vi "Dashboard Main.vi"() -> ()   [LabVIEW 2020]
uses:
  <vilib>/event_ctls.llb/eventvkey.ctl
  <vilib>/Rock Robotics/Network Tables/NT Read Numeric Array.vi
  <vilib>/Rock Robotics/Network Tables/NT Read Boolean.vi
  <vilib>/Rock Robotics/WPI/Dashboard/WPI_DashboardLogging Global.vi
panel:
  in  "Camera Settings Right":T1={"Frame Rate"=30, "Compression"=30, "Size"=1, "DB Camera Config"=FALSE} {"Frame Rate" scale=1.0..30.0; "Compression" scale=100.0..-1.0; "Size" items=["640x480", "320x240", "160x120"]}
  in  "Camera Name Right":string(combo)="No Camera Selection"
  out "Camera Perf":string
  in  "Camera Settings":T1={"Frame Rate"=30, "Compression"=30, "Size"=1, "DB Camera Config"=FALSE} {"Frame Rate" scale=1.0..30.0; "Compression" scale=100.0..-1.0; "Size" items=["640x480", "320x240", "160x120"]}
  in  "TCP":refnum<k5>
  in  "Rec Mode":enum32{"Stop", "Record", "Playback"}(radio)
  out "Robot IP":string
  out "Image Message":string="Timeout in Camera Communications"
  in  "Dashboard Tab":T2(tab)
  out "Reverse":bool
  out "Speed Modifer":dbl
  in  "Select Auto":string(combo)="Select Autonomous ..."
  out "NT Connection":bool
  out "JS1 Z":dbl(slide) scale=-1.0..1.0 scale format="%#_2e"
  out "JS1 Graph":cluster{"X":dbl, "Y":dbl}[](graph)
  out "JS1 Buttons":T3
  out "JS2 Z":dbl(slide) scale=-1.0..1.0 scale format="%#_2e"
  out "JS2 Graph":cluster{"X":dbl, "Y":dbl}[](graph)
  out "JS2 Buttons":T3
  out "Mode":T4(ring)=enum."Auto Disabled"
  out "Right Camera Perf":cluster{"Bandwidth (Mbps)":dbl, "FPS":dbl}
  out "Camera Image Right":T5(plugin-control)
  in  "DB/String 9":string
  in  "DB/String 8":string
  in  "DB/String 7":string
  in  "DB/String 6":string
  in  "DB/String 5":string
  in  "DB/String 4":string
  in  "DB/String 3":string
  in  "DB/String 2":string
  in  "DB/String 1":string
  in  "DB/String 0":string
  in  "DB/Slider 0":dbl(slide) scale=0.0..5.0
  in  "DB/Slider 1":dbl(slide) scale=0.0..5.0
  in  "DB/Slider 2":dbl(slide) scale=0.0..5.0
  in  "DB/Slider 3":dbl(slide) scale=0.0..5.0
  out "DB/LED 3":bool
  out "DB/LED 2":bool
  out "DB/LED 1":bool
  out "DB/LED 0":bool
  in  "DB/Button 3":bool
  in  "DB/Button 2":bool
  in  "DB/Button 1":bool
  in  "DB/Button 0":bool caption="New Name"
  in  "Test Slider":dbl(slide) scale=0.0..100.0 scale format="%#_3g"
  in  "On/Off":bool caption="Solenoid"
  in  "Test Name":u16(ring) items=["Select the test to run..."]
  in  "Test Tree":string(tree)
  in  "Motor":cluster{"Value":dbl, "Enable":bool} {"Value" scale=-1.0..1.0 scale format="%#_3g"}
  out "Progress":T6 {"Test Progress" scale=0.0..100.0}
  in  "Rev/Fwd":cluster{"Forward":bool, "Reverse":bool}
  in  "Test Ring":u16(ring) items=["Monochrome", "Color"]
  in  "CheckList":i32(listbox)
  out "Tree":string(tree)
  out "Camera Image":T5(plugin-control)
  out "Background":bool
  in  "Camera Name":string(combo)="No Camera Selection"
  # "HW"
  # "HW"
  # "Joysticks"
  # "This tab is a great place for autonomous settings and robot-specific values.\nPlace controls and indicators inside this tab and match name to\nDashboard Variables on robot. You can also delete this comment."
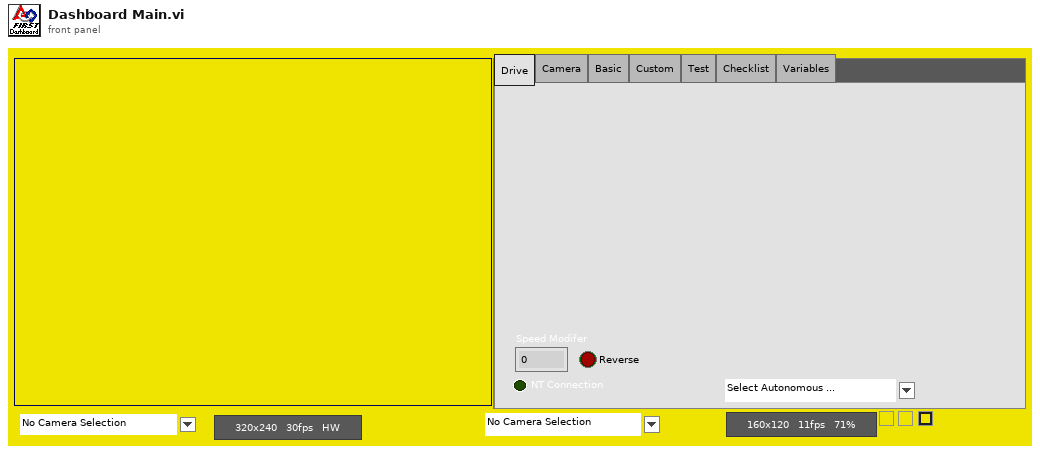
[diagram p1: front panel]
types:
  T1 = cluster{"Frame Rate":i32, "Compression":i32, "Size":u16, "DB Camera Config":bool}
  T2 = enum32{"Drive", "Camera", "Basic", "Custom", "Test", "Checklist", "Variables"}
  T3 = cluster{bool, bool, bool, bool, bool, bool, bool, bool, bool, bool, bool, bool}
  T4 = enum8{"Tele-Op Disabled", "Tele-Op Enabled", "Auto Disabled", "Auto Enabled", "Test Disabled", "Test Enabled", "Disconnected", "No Code", "E-Stop"}
  T5 = typedef "IMAQ Image.ctl" = refnum<image>
  T6 = cluster{"Test Progress":u8, "Test Progress Text":string}
  T7 = cluster{"Save Path":path, "Interval (s)":dbl, "Keep":i32}
  T8 = enum32{"Drive", "Camera", "Basic", "Custom", "Test", "Commands", "Checklist", "Variables"}
  T9 = typedef "Image Type" = u32
  T10 = cluster{"Error Strings":string, "Disable Counts":cluster{u16, u16}, "Rail Faults":cluster{u16, u16, u16}, "Robot IP":string, "DB Mode":u8, "Event Info":cluster{"Name":string, "Type":u8, "Number":u16, "Replay":u8}}
  T11 = cluster{"Storage":cluster{"Disk Free":u64, "RAM Block":u32, "RAM free":u32}, "CPU Utilization":cluster{"CPU % ISR":sgl, "CPU % Time Crit":sgl, "CPU % Timed Str":sgl, "CPU % High":sgl, "CPU % Above":sgl, "CPU % Normal":sgl, "CPU % Low":sgl}, "CAN":cluster{"% Bus Utilization":sgl, "Bus Off Cnt":u32, "TX_FIFO Full Cnt":u32, "Receive Error Cnt":u8, "Transmit Error Cnt":u8}, "HID":cluster{"HID Outputs":u32, "Rumble Low":u16, "Rumble High":u16}[]}
  T12 = cluster{"Status bits":cluster{"Test Mode":bool, "Autonomous":bool, "Enabled":bool, "Code Start":bool, "Brownout":bool, "Reserved 2":bool, "Reserved 3":bool, "E-Stop":bool}, "Code Trace":cluster{"Disabled":bool, "TeleOp":bool, "Auto":bool, "Test":bool}, "Controller Type":enum16{"unknown", "cRIO", "roboRio"}, "Code?":enum16{"unknown", "noCode", "code"}, "Battery V":dbl}
  T13 = cluster{"Control Bits":cluster{"TestMode":bool, "Autonomous":bool, "Enabled":bool, "FMS Present":bool, bool, bool, bool, "E-Stop":bool}, "Team Station ":u8, "Countdown":sgl, "Joystick Values":cluster{"Axes":dbl[], "Buttons":bool[], "POVs":i16[]}[]}
  T14 = cluster{"Axes":dbl[], "Buttons":bool[], "POVs":i16[]}[]
  T15 = cluster{"Axes":dbl[], "Buttons":bool[], "POVs":i16[]}
  T16 = cluster{"Buttons[0]":bool, "Buttons[1]":bool, "Buttons[2]":bool, "Buttons[3]":bool, "Buttons[4]":bool, "Buttons[5]":bool, "Buttons[6]":bool, "Buttons[7]":bool, "Buttons[8]":bool, "Buttons[9]":bool, "Buttons[10]":bool, "Buttons[11]":bool}
  T17 = cluster{"Camera Image":refnum<vi>, "Dashboard Tab":refnum<vi>, "Background":refnum<vi>, "Rec Mode":refnum<vi>, "Test Slider":refnum<vi>, "On/Off ":refnum<vi>, "Test Ring":refnum<vi>, "Rev/Fwd":refnum<vi>, "Test Name":refnum<vi>, "Motor":refnum<vi>, "Progress":refnum<vi>, "CheckList":refnum<vi>, "Tree":refnum<vi>, "Test Tree":refnum<vi>, "Camera Settings":refnum<vi>, "Camera Name":refnum<vi>, "Camera Perf":refnum<vi>, "Camera Settings Right":refnum<vi>, "Camera Name Right":refnum<vi>, "Camera Image Right":refnum<vi>}
  T18 = cluster{"Global Rectangle":i32[], "Contours":cluster{"Contour Type":u32, "ROI Type":u32, "Points":i32[]}[]}
  T19 = cluster{"Camera Name":string, string, "Saved DB Images Info":cluster{"Save Path":path, "Interval (s)":dbl, "Keep":i32}}
  T20 = cluster{"Camera Name Right":string, string, "Saved DB Images Info":cluster{"Save Path":path, "Interval (s)":dbl, "Keep":i32}}
  T21 = cluster{"Operation":enum16{"Update", "Clear"}, "Color Box":u32}[]
  T22 = typedef "eventvkey.ctl" = enum16{"ASCII", "Enter", "Return", "Shift", "Ctrl", "Alt", "Cmd", "Opt", "Caps", "NumLock", "Clear", "Break", "Up", "Down", "Left", "Right", "Insert", "Delete", "Home", "End", "PageUp", "PageDown", "Escape", "Help", "Pause", "ScrollLock", "F1", "F2", "F3", "F4", "F5", "F6", "F7", "F8", "F9", "F10", "F11", "F12", "F13", "F14", "F15", "F16", "F17", "F18", "F19", "F20", "F21", "F22", "F23", "F24", "Play", "VolumeUp", "VolumeDown", "Mute", "Two Byte Char"}
  T23 = cluster{"Image Size":bool, "Image Type":bool, "Pixel Value":bool, "ROI Information":bool, "Zoom Factor":bool}
  T24 = cluster{"Operation":enum16{"Update", "Clear"}, "Color Box":u32}
  T25 = cluster{"Shift":bool, "Ctrl":bool, "Alt":bool, "Cmd":bool, "Opt":bool}
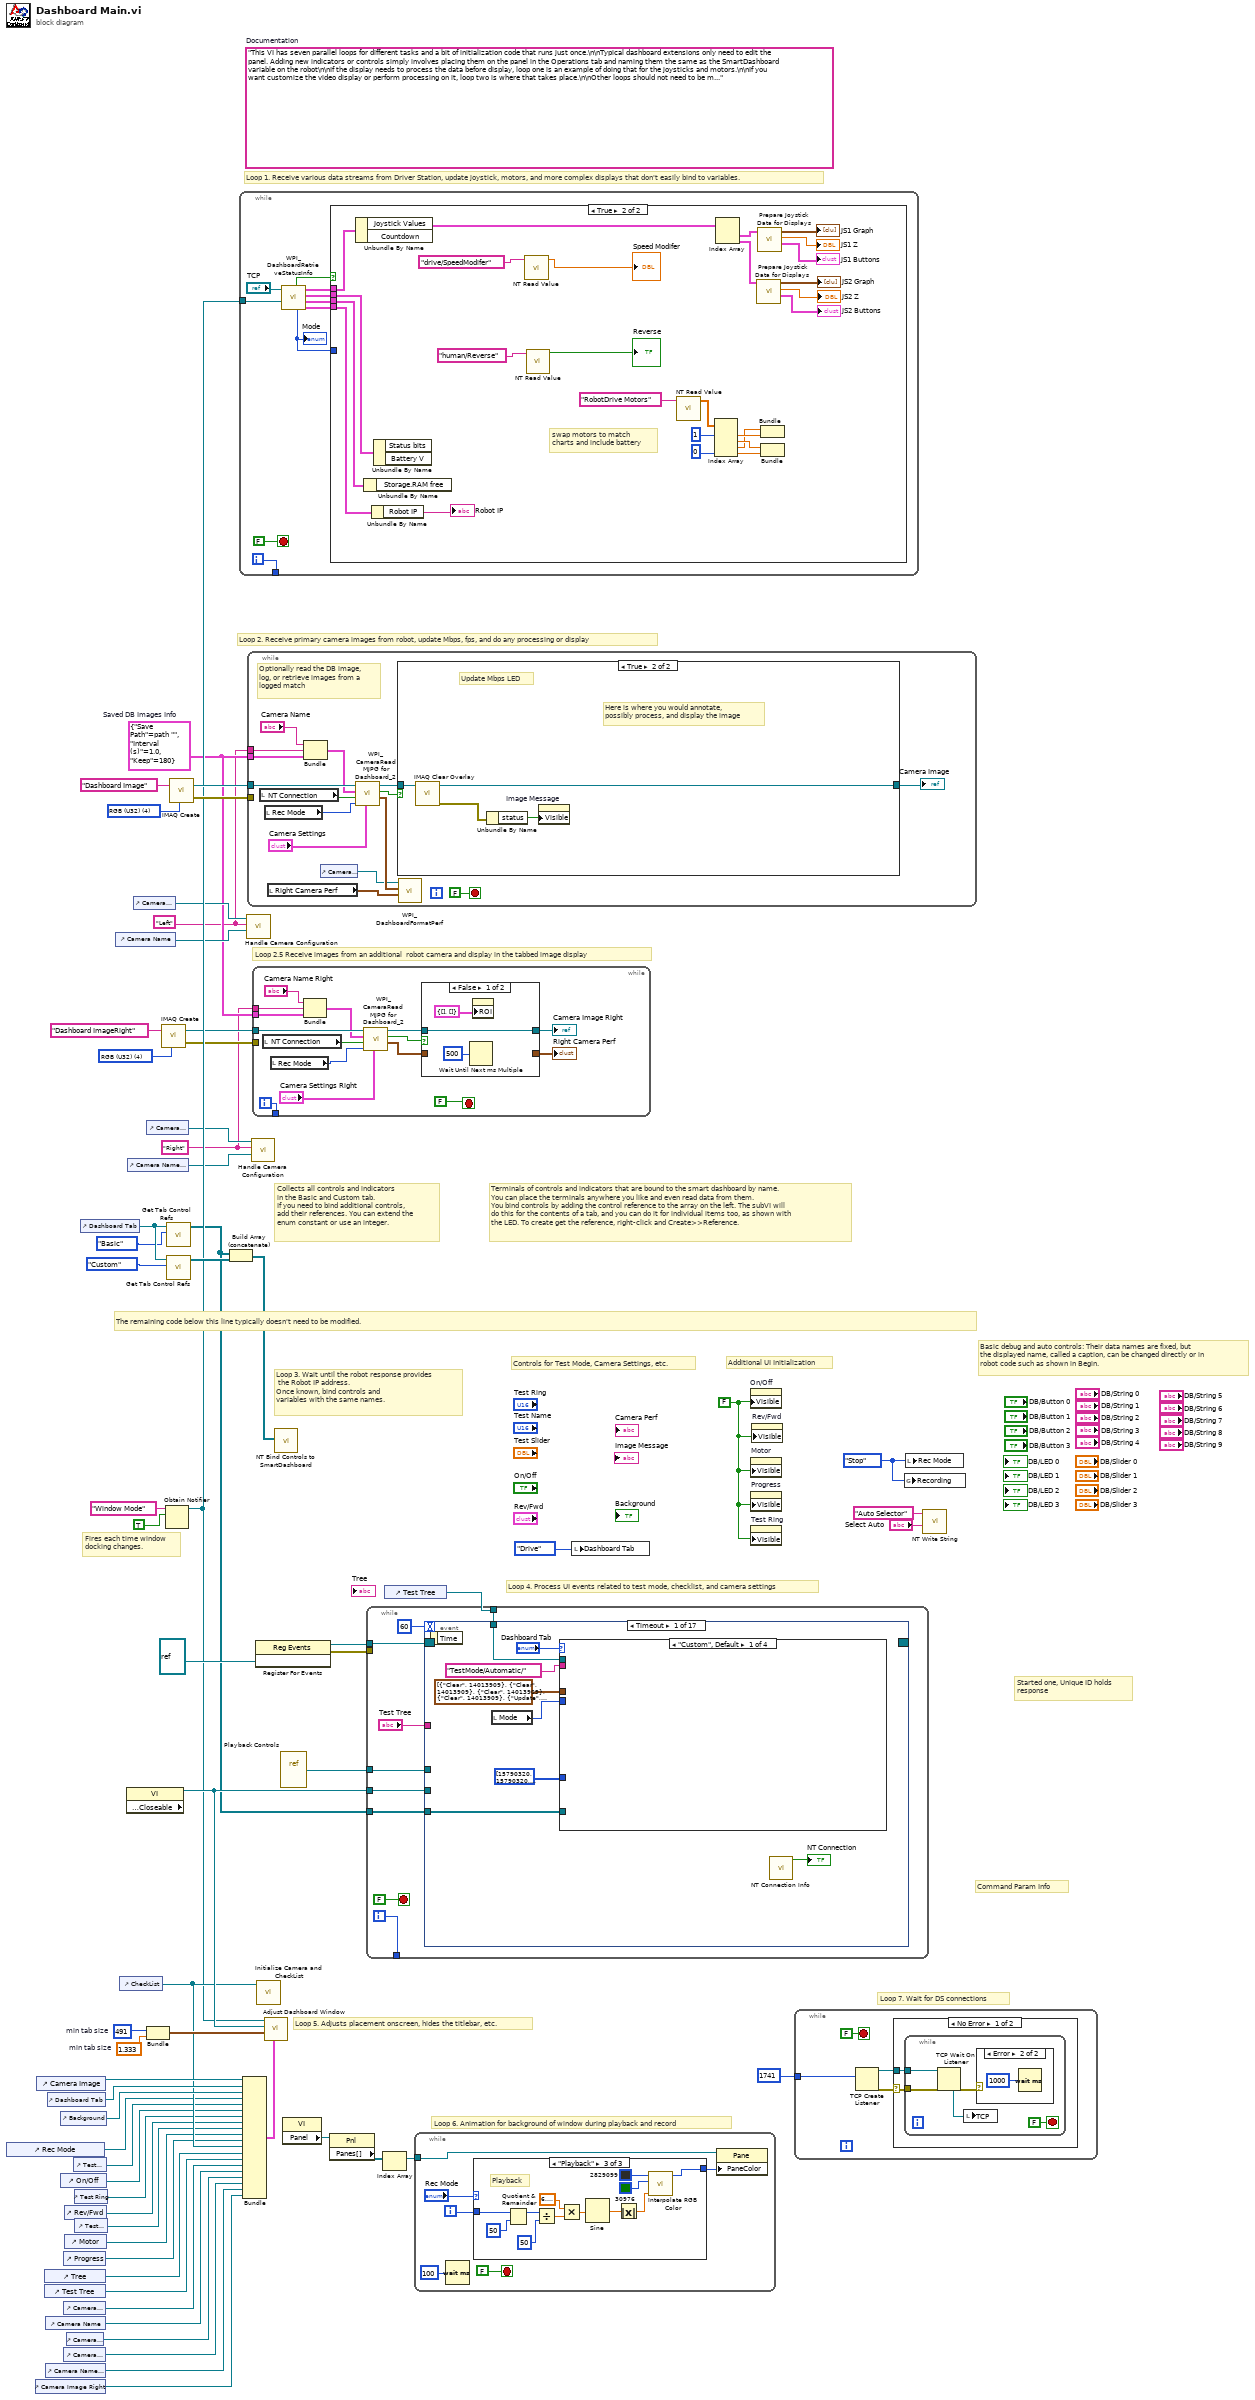
[diagram p0: block diagram]
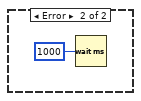
[diagram p4: hidden frame]
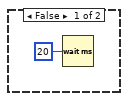
[diagram p5: hidden frame]
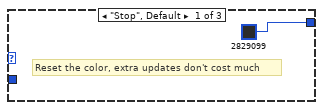
[diagram p6: hidden frame]
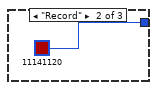
[diagram p7: hidden frame]
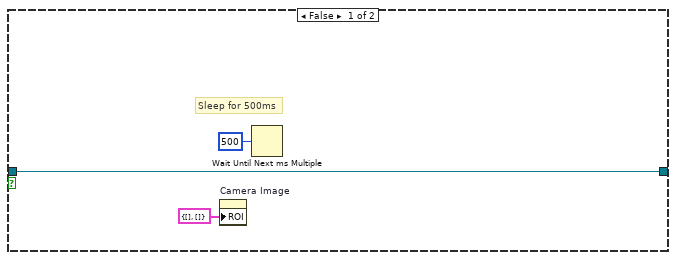
[diagram p8: hidden frame]
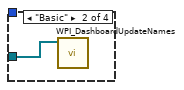
[diagram p9: hidden frame]
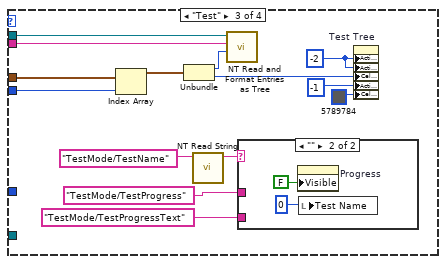
[diagram p10: hidden frame]
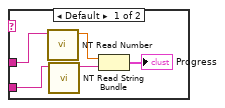
[diagram p11: hidden frame]
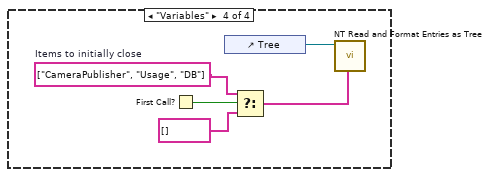
[diagram p12: hidden frame]
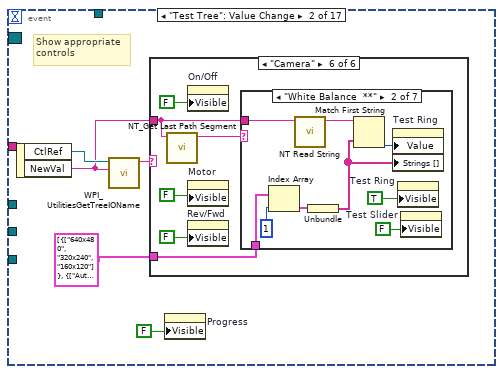
[diagram p13: hidden frame]
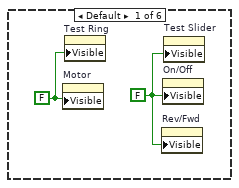
[diagram p14: hidden frame]
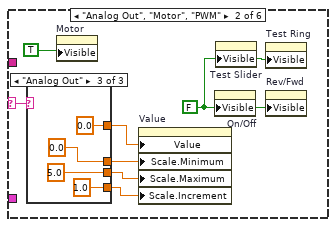
[diagram p15: hidden frame]
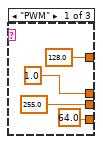
[diagram p16: hidden frame]
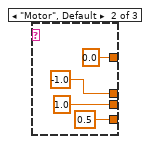
[diagram p17: hidden frame]
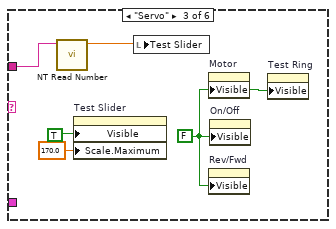
[diagram p18: hidden frame]
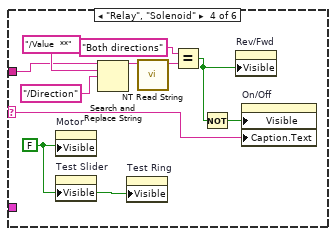
[diagram p19: hidden frame]
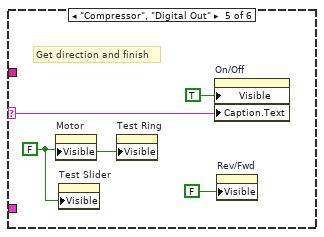
[diagram p20: hidden frame]
diagram:
  w3 = T7 {"Save Path"=path "", "Interval (s)"=1.0, "Keep"=180}  # Saved DB Images Info
  w2 = "Right"
  w1 = "Left"
  w13 = T9 4 items=["Grayscale (U8)", "Grayscale (I16)", "Grayscale (SGL)", "Complex (CSG)", "RGB (U32)", "HSL (U32)", "RGB (U64)"] ("Image Type")
  w42 = 491  # min tab size
  w41 = 1.333  # min tab size
  w49 = enum32{"Stop", "Record", "Playback"}."Stop" ("Rec Mode")
  w26 = FALSE ("Visible")
  (unwired) "This VI has seven parallel loops for different tasks and a bit of initialization code that runs just once.\n\nTypical dashboard extensions only need to edit the panel. Adding new indicators or controls simply involves placing them on the panel in the Operations tab and naming them the same as the SmartDashboard variable on the robot\n\nIf the display needs to process the data before display, loop one is an example of doing that for the joysticks and motors.\n\nIf you want customize the video display or perform processing on it, loop two is where that takes place.\n\nOther loops should not need to be modified. They are pretty standard, and document the task they perform."  # Documentation
  w63 = T9 4 items=["Grayscale (U8)", "Grayscale (I16)", "Grayscale (SGL)", "Complex (CSG)", "RGB (U32)", "HSL (U32)", "RGB (U64)"] ("Image Type")
  # "Loop 2.5 Receive images from an additional  robot camera and display in the tabbed image display"
  # "Command Param Info"
  # "Started one, Unique ID holds\nresponse"
  # "Loop 7. Wait for DS connections"
  # "Basic debug and auto controls: Their data names are fixed, but\nthe displayed name, called a caption, can be changed directly or in\nrobot code such as shown in Begin."
  # "Controls for Test Mode, Camera Settings, etc."
  # "Additional UI Initialization"
  # "Loop 6. Animation for background of window during playback and record"
  # "Fires each time window\ndocking changes."
  # "Collects all controls and indicators\nin the Basic and Custom tab.\nIf you need to bind additional controls,\nadd their references. You can extend the\nenum constant or use an integer."
  # "The remaining code below this line typically doesn't need to be modified."
  # "Loop 4. Process UI events related to test mode, checklist, and camera settings"
  # "Terminals of controls and indicators that are bound to the smart dashboard by name.\nYou can place the terminals anywhere you like and even read data from them.\nYou bind controls by adding the control reference to the array on the left. The subVI will\ndo this for the contents of a tab, and you can do it for individual items too, as shown with\nthe LED. To create get the reference, right-click and Create>>Reference."
  # "Loop 3. Wait until the robot response provides\n the Robot IP address.\nOnce known, bind controls and\nvariables with the same names."
  # "Loop 5. Adjusts placement onscreen, hides the titlebar, etc."
  # "Loop 1. Receive various data streams from Driver Station, update joystick, motors, and more complex displays that don't easily bind to variables."
  # "Loop 2. Receive primary camera images from robot, update Mbps, fps, and do any processing or display"
  n1 = control-ref of="Rec Mode"() -> (w32:refnum<vi>)
  n2 = control-ref of="Camera Image Right"() -> (w6:refnum<vi>)
  n3 = control-ref of="Camera Image"() -> (w44:refnum<vi>)
  n4 = control-ref of="Tree"() -> (w36:refnum<vi>)
  n5 = control-ref of="Test Tree"() -> (w35:refnum<vi>)
  n6 = control-ref of="Camera Name"() -> (w19:refnum<vi>)
  n7 = control-ref of="Camera Name Right"() -> (w7:refnum<vi>)
  n8 = control-ref of="Dashboard Tab"() -> (w43:refnum<vi>)
  n9 = control-ref of="Background"() -> (w39:refnum<vi>)
  n10 = control-ref of="On/Off"() -> (w30:refnum<vi>)
  n11 = control-ref of="Progress"() -> (w27:refnum<vi>)
  n12 = control-ref of="Camera Settings"() -> (w20:refnum<vi>)
  n13 = control-ref of="Camera Settings Right"() -> (w8:refnum<vi>)
  n14 = control-ref of="Rev/Fwd"() -> (w28:refnum<vi>)
  n15 = control-ref of="Motor"() -> (w33:refnum<vi>)
  n16 = control-ref of="Camera Perf"() -> (w18:refnum<vi>)
  n17 = control-ref of="Test Slider"() -> (w31:refnum<vi>)
  n18 = control-ref of="Test Ring"() -> (w29:refnum<vi>)
  n19 = control-ref of="Test Name"() -> (w34:refnum<vi>)
  n20 = control-ref of="Dashboard Tab"() -> (w47:refnum<vi>)
  n21 = control-ref of="Camera Name"() -> (w21:refnum<vi>)
  n22 = control-ref of="CheckList"() -> (w37:refnum<vi>)
  n23 = property class="VI" props=["Front Panel.Closeable"]() -> (reference out=w48:refnum<vi>)  [unwired: 2 in, 2 out]
  n24 = control-ref of="Camera Name Right"() -> (w9:refnum<vi>)
  n25 = control-ref of="Camera Settings"() -> (w22:refnum<vi>)
  n26 = control-ref of="Camera Settings Right"() -> (w10:refnum<vi>)
  n27 = Bundle("min tab size"=w42, "min tab size"=w41) -> (w40:cluster{"min tab size":i32, "min tab size":dbl})  [unwired: 1 in]
  n28 = call "IMAQ Create"("Image Name"="Dashboard ImageRight", "Image Type"=w13) -> ("New Image"=w12:T5, "error out"=w11:errorcluster)  [unwired: 2 in, 1 out]
  n29 = Obtain Notifier(name (unnamed)="Window Mode", notification data type=TRUE) -> (notifier out=w25:refnum<notifier>)  [unwired: 2 in, 2 out]
  n30 = call <vilib>:"Get Tab Control Refs.vi"("Page Index"=T8."Basic" ("Dashboard Tab"), "TabControl in"=w47) -> ("ControlsOnPage"=w17:refnum<vi>[])  [unwired: 9 in]
  n31 = call <vilib>:"Get Tab Control Refs.vi"("Page Index"=T8."Custom" ("Dashboard Tab"), "TabControl in"=w47) -> ("ControlsOnPage"=w46:refnum<vi>[])  [unwired: 9 in]
  n32 = call "IMAQ Create"("Image Name"="Dashboard Image", "Image Type"=w63) -> ("New Image"=w61:T5, "error out"=w60:errorcluster)  [unwired: 2 in, 1 out]
  n33 = Build Array (concatenate)(w17, w46) -> (w45:refnum<vi>[])
  n34 = while {
    tunnel: [w72] -> _
    tunnel: w25 -> [w64]
    i -> [w72]
    stop <- FALSE stop-if-true
    n35 = call <vilib>:"WPI_DashboardRetrieveStatusInfo.vi"("Window Mode Notifier"=w64, "TCP Cnx"="TCP") -> ("Power and Errors"=w67:T10, "Robot Metrics"=w70:T11, "Status Info"=w71:T12, "Control Info"=w68:T13, "Robot Mode"=w66:T4, "Process?"=w69:bool)  [unwired: 4 in]
    "Mode" <- w66
    n36 = case shown="True" w69 {
      tunnel: w71 -> [_ w100]
      tunnel: w70 -> [_ w99]
      tunnel: w68 -> [_ w98]
      tunnel: w67 -> [_ w97]
      tunnel: w66 -> [_ _]
      frame False {
        n37 = Wait (ms)(milliseconds to wait=u32 20) -> ()  [unwired: 1 out]
      }
      frame True {
        # "swap motors to match\ncharts and include battery"
        n38 = Unbundle By Name(w98) -> ("Joystick Values"=w90:T14)  [unwired: 1 out]
        n39 = Unbundle By Name(w99) -> ()  [unwired: 1 out]
        n40 = Unbundle By Name(w97) -> ("Robot IP"=→"Robot IP":string)
        n41 = Unbundle By Name(w100) -> ()  [unwired: 2 out]
        n42 = call-poly <vilib>:"NT Read Value.vi"("name"="drive/SpeedModifer") -> ("value"=→"Speed Modifer":dbl)  [unwired: 8 in, 2 out]
        n43 = call-poly <vilib>:"NT Read Value.vi"("name"="human/Reverse") -> ("value"=→"Reverse":bool)  [unwired: 8 in, 2 out]
        n44 = call-poly <vilib>:"NT Read Value.vi"("name"="RobotDrive Motors" ("Name")) -> ("value"=w80:dbl[])  [unwired: 8 in, 2 out]
        n45 = Index Array(array=w80, index #1=1, index #4=0) -> (element #1=w92:dbl, element #2=w93:dbl, element #3=w91:dbl, element #4=w96:dbl)  [unwired: 2 in]
        n46 = Index Array(array=w90) -> (element #1=w89:T15, element #2=w85:T15)  [unwired: 2 in]
        n47 = call "Prepare Joystick Data for Displays.vi"("Joystick Values"=w85) -> ("Buttons"=→"JS2 Buttons":T16, "Z Axis"=→"JS2 Z":dbl, "Cartesian Data"=→"JS2 Graph":cluster{"X axis":dbl, "X axis":dbl}[])  [unwired: 8 in]
        n48 = call "Prepare Joystick Data for Displays.vi"("Joystick Values"=w89) -> ("Buttons"=→"JS1 Buttons":T16, "Z Axis"=→"JS1 Z":dbl, "Cartesian Data"=→"JS1 Graph":cluster{"X axis":dbl, "X axis":dbl}[])  [unwired: 8 in]
        n49 = Bundle("Numeric"=w91, "Numeric"=w92) -> ()  [unwired: 1 in, 1 out]
        n50 = Bundle("Numeric"=w93, "Numeric"=w96) -> ()  [unwired: 1 in, 1 out]
      }
    }
  }
  n51 = Bundle("Camera Image"=w44, "Dashboard Tab"=w43, "Background"=w39, "Rec Mode"=w32, "Test Slider"=w31, "On/Off"=w30, "Test Ring"=w29, "Rev/Fwd"=w28, "Test Name"=w34, "Motor"=w33, "Progress"=w27, "CheckList"=w37, "Tree"=w36, "Test Tree"=w35, "Camera Settings"=w20, "Camera Name"=w19, "Camera Perf"=w18, "Camera Settings Right"=w8, "Camera Name Right"=w7, "Camera Image Right"=w6) -> (w38:T17)  [unwired: 1 in]
  n52 = call "Handle Camera Configuration.vi"("CameraNameRef"=w21, "Display Name"=w1, "ClusterRef"=w22) -> ()  [unwired: 9 in]
  n53 = while {
    tunnel: w61 -> [w114]
    tunnel: w60 -> [_]
    tunnel: w3 -> [w107]
    tunnel: w1 -> [w104]
    stop <- FALSE stop-if-true
    # "Optionally read the DB image,\nlog, or retrieve images from a\nlogged match"
    n54 = local read "NT Connection"() -> (w108:bool)
    n55 = local read "Rec Mode"() -> (w111:enum32{"Stop", "Record", "Playback"})
    n56 = local read "Right Camera Perf"() -> (w102:cluster{"Bandwidth (Mbps)":dbl, "FPS":dbl})
    n57 = Bundle("Camera Name"="Camera Name", w104, "Saved DB Images Info"=w107) -> (w106:T19)  [unwired: 1 in]
    n58 = control-ref of="Camera Perf"() -> (w101:refnum<vi>)
    n59 = call <vilib>:"WPI_CameraRead MJPG for Dashboard_2.vi"("Camera Settings"="Camera Settings", "Rec Mode"=w111, "NT Connection"=w108, "Capture Info"=w106, "Image in"=w114) -> ("perf info"=w103:cluster{"Bandwidth (Mbps)":dbl, "fps":dbl}, "Active"=w112:bool, "Image\\ out"=w113:T5)  [unwired: 4 in]
    n60 = case shown="True" w112 {
      tunnel: w113 -> [w117 w120]
      tunnel: [w117 w119] -> w109
      frame False {
        # "Sleep for 500ms"
        n61 = property on="Camera Image" class="ImageControl"("ROI"=T18 {"Global Rectangle"=[], "Contours"=[]}) -> ()  [unwired: 2 in, 2 out]
        n62 = Wait Until Next ms Multiple(millisecond multiple=u32 500) -> ()  [unwired: 1 out]
      }
      frame True {
        # "Here is where you would annotate,\npossibly process, and display the image"
        # "Update Mbps LED"
        n63 = call "IMAQ Clear Overlay"("Image"=w120) -> ("error out"=w121:errorcluster, "Image Out"=w119:T5)  [unwired: 2 in, 7 out]
        n64 = Unbundle By Name(w121) -> ("status"=w122:bool)
        n65 = property on="Image Message" class="Str"("Visible"=w122) -> ()  [unwired: 2 in, 2 out]
      }
    }
    "Camera Image" <- w109
    n66 = call <vilib>:"WPI_DashboardFormatPerf.vi"("Right Camera Perf"=w102, "Performance"=w103, "String in"=w101) -> ()  [unwired: 9 in]
  }
  n67 = call "Handle Camera Configuration.vi"("CameraNameRef"=w9, "Display Name"=w2, "ClusterRef"=w10) -> ()  [unwired: 9 in]
  n68 = while {
    tunnel: w12 -> [w137]
    tunnel: w11 -> [_]
    tunnel: [w132] -> _
    tunnel: w3 -> [w128]
    tunnel: w2 -> [w125]
    i -> [w132]
    stop <- FALSE stop-if-true
    n69 = local read "NT Connection"() -> (w129:bool)
    n70 = local read "Rec Mode"() -> (w136:enum32{"Stop", "Record", "Playback"})
    n71 = Bundle("Camera Name Right"="Camera Name Right", w125, "Saved DB Images Info"=w128) -> (w127:T20)  [unwired: 1 in]
    n72 = call <vilib>:"WPI_CameraRead MJPG for Dashboard_2.vi"("Camera Settings"="Camera Settings Right", "Rec Mode"=w136, "NT Connection"=w129, "Capture Info"=w127, "Image in"=w137) -> ("perf info"=w123:cluster{"Bandwidth (Mbps)":dbl, "fps":dbl}, "Active"=w131:bool, "Image\\ out"=w134:T5)  [unwired: 4 in]
    n73 = case shown="False" w131 {
      tunnel: w134 -> [w139 w142]
      tunnel: [w139 w142] -> w130
      tunnel: [_ w141] -> w124
      tunnel: w123 -> [_ w141]
      frame False {
        n74 = Wait Until Next ms Multiple(millisecond multiple=u32 500) -> ()  [unwired: 1 out]
        n75 = property on="Camera Image Right" class="ImageControl"("ROI"=T18 {"Global Rectangle"=[], "Contours"=[]}) -> ()  [unwired: 2 in, 2 out]
      }
      frame True {
      }
    }
    "Camera Image Right" <- w130
    "Right Camera Perf" <- w124
  }
  n76 = register-events(refnum<vi> refnum) -> (reference out=w52:refnum<event-registration>, error out=w51:errorcluster)  [unwired: 2 in]
  n77 = call "Initialize Camera and CheckList.vi"("ListBox in"=w37) -> ()  [unwired: 11 in]
  n78 = call "Adjust Dashboard Window.vi"("Sizing Refnums"=w38, "Size Constraints"=w40, "VI"=w48, "WIn Mode"=w25) -> ()  [unwired: 8 in]
  n79 = call <vilib>:"NT Bind Controls to SmartDashboard.vi"("Bound Control Refs"=w45) -> ()  [unwired: 11 in]
  n80 = vi-ref "Playback Controls.vi"() -> (w53:refnum<vi>)
  n81 = property class="VI"() -> ("Panel"=w55:refnum<vi>)  [unwired: 2 in, 2 out]
  n82 = property class="Pnl"(reference=w55) -> ("Panes[]"=w56:refnum<vi>[])  [unwired: 1 in, 2 out]
  n83 = Index Array(array=w56) -> (element=w54:refnum<vi>)  [unwired: 1 in]
  n84 = control-ref of="Test Tree"() -> (w57:refnum<vi>)
  n85 = while {
    tunnel: [w148] -> _
    tunnel: w57 -> [w147]
    tunnel: w53 -> [w146]
    tunnel: w52 -> [w145]
    tunnel: w51 -> [_]
    tunnel: w48 -> [w144]
    tunnel: w17 -> [w143]
    i -> [w148]
    stop <- FALSE stop-if-true
    n86 = event shown="[0] Timeout" {
      selector: w145 -> [_ _ _ _ _ _ _ _ _ _ _ _ _ _ _ _ _]
      dyn-events: [_ _ _ _ _ _ _ _ _ _ _ _ _ w353 _ _ _] -> _
      timeout: u32 60 ("milliseconds to wait") -> [_ _ _ _ _ _ _ _ _ _ _ _ _ _ _ _ _]
      tunnel: w147 -> [w158 _ _ _ _ _ _ _ _ _ _ _ _ _ _ _ _]
      tunnel: "Test Tree" -> [_ _ _ _ _ _ _ _ w326 w333 w334 w337 w344 _ _ _ _]
      tunnel: w146 -> [_ _ _ _ _ _ _ _ _ _ _ _ _ w355 _ w370 _]
      tunnel: w144 -> [_ _ _ _ _ _ _ _ _ _ _ _ _ w351 _ _ _]
      tunnel: w143 -> [w153 _ _ _ _ _ _ _ _ _ _ _ _ _ _ _ _]
      event Timeout {
        n87 = event-data() -> ()  [unwired: 1 in, 1 out]
        n88 = local read "Mode"() -> (w156:T4)
        n89 = case shown="\"Custom\", Default" "Dashboard Tab" {
          tunnel: w158 -> [_ _ w174 _]
          tunnel: "TestMode/Automatic/" ("Name Pattern") -> [_ _ w173 _]
          tunnel: T21 [{"Operation"=enum."Clear", "Color Box"=14013909}, {"Operation"=enum."Clear", "Color Box"=14013909}, {"Operation"=enum."Clear", "Color Box"=14013909}, {"Operation"=enum."Clear", "Color Box"=14013909}, {"Operation"=enum."Update", "Color Box"=14013909}, {"Operation"=enum."Update", "Color Box"=16777215}, {"Operation"=enum."Clear", "Color Box"=14013909}, {"Operation"=enum."Clear", "Color Box"=14013909}, {"Operation"=enum."Clear", "Color Box"=14013909}] -> [_ _ w166 _]
          tunnel: w156 -> [_ _ w165 _]
          tunnel: u32[] [15790320, 15790320, 15790320, 15790320, 16777215, 16777215, 15790320, 15790320, 15790320] -> [_ _ _ _]
          tunnel: w153 -> [_ w160 _ _]
          frame "Custom", Default {
          }
          frame "Basic" {
            n90 = call <vilib>:"WPI_DashboardUpdateNames.vi"("Controls on Tab"=w160) -> ()  [unwired: 11 in]
          }
          frame "Test" {
            w172 = -2 ("Active Item:Row Number")
            n91 = Index Array(array=w166, index=w165) -> (element=w167:T24)
            n92 = Unbundle(w167) -> ("Operation"=w168:enum16{"Update", "Clear"}, "Color Box"=w169:u32)
            n93 = call <vilib>:"NT Read String.vi"("name"="TestMode/TestName" ("Name")) -> ("value"=w163:string)  [unwired: 8 in, 2 out]
            n94 = call <vilib>:"NT Read and Format Entries as Tree.vi"("Operation"=w168, "Name Pattern"=w173, "Tree Refnum"=w174) -> ()  [unwired: 7 in, 2 out]
            n95 = case shown="\"\"" w163 {
              tunnel: "TestMode/TestProgress" ("Name") -> [w176 _]
              tunnel: "TestMode/TestProgressText" ("Name") -> [w175 _]
              frame Default {
                n96 = call <vilib>:"NT Read Number.vi"("name"=w176) -> ("value"=w177:dbl)  [unwired: 8 in, 2 out]
                n97 = call <vilib>:"NT Read String.vi"("name"=w175) -> ("value"=w178:string)  [unwired: 8 in, 2 out]
                n98 = Bundle("value"=w177, "value"=w178) -> (→"Progress":cluster{"value":dbl, "value":string})  [unwired: 1 in]
              }
              frame "" {
                n99 = property on="Progress" class="Clust (strict)"("Visible"=FALSE) -> ()  [unwired: 2 in, 2 out]
                n100 = local write "Test Name"(u16 0) -> ()
              }
            }
            n101 = property on="Test Tree" class="Tree (strict)"("Active Item Row Number"=w172, "ActiveColNum"=w172, "CellBG"=w169, "Active Item Row Number"=-1 ("Active Item:Row Number"), "CellBG"=u32 5789784 ("Color Box")) -> ()  [unwired: 2 in, 2 out]
          }
          frame "Variables" {
            w184 = string[] ["CameraPublisher", "Usage", "DB"]  # Items to initially close
            n102 = First Call?() -> (First Call?: T/F=w185:bool)
            n103 = control-ref of="Tree"() -> (w186:refnum<vi>)
            n104 = Select(t=w184, s=w185, f=string[] []) -> (s? t:f=w182:string[])
            n105 = call <vilib>:"NT Read and Format Entries as Tree.vi"("Tags to  Close"=w182, "Tree Refnum"=w186) -> ()  [unwired: 8 in, 2 out]
          }
        }
        n106 = call <vilib>:"NT Connection Info.vi"() -> ("Connected"=→"NT Connection":bool)  [unwired: 11 in]
      }
      event "Test Tree": Value Change {
        # "Show appropriate\ncontrols"
        n107 = event-data() -> ("CtlRef"=w190:refnum<vi>, "NewVal"=w188:string)  [unwired: 1 in]
        n108 = call <vilib>:"WPI_UtilitiesGetTreeIOName.vi"("NewVal"=w188, "TreeControl in"=w190) -> ("I/O Name"=w191:string)  [unwired: 9 in]
        n109 = case shown="\"Camera\"" w191 {
          selector: w191 -> [_ w198 _ w220 w229 _]
          tunnel: w188 -> [_ _ w217 w219 _ w236]
          tunnel: cluster{string[]}[] [{["640x480", "320x240", "160x120"]}, {["Auto", "Fixed indoor", "Fixed outdoor 1", "Fixed outdoor 2", "Fixed fluorescent 1", "Fixed fluorescent 2", "Hold current"]}, {["Auto", "Flicker-free 50 Hz", "Flicker-free 60 Hz", "Hold current"]}, {["None", "Prioritize frame rate", "Prioritize image quality"]}, {["Monochrome", "Color"]}] -> [_ _ _ _ _ w235]
          frame Default {
            w193 = FALSE ("Visible")
            w192 = FALSE ("Visible")
            n110 = property on="Motor" class="Clust (strict)"("Visible"=w192) -> ()  [unwired: 2 in, 2 out]
            n111 = property on="Test Ring" class="Ring (strict)"("Visible"=w192) -> ()  [unwired: 2 in, 2 out]
            n112 = property on="Rev/Fwd" class="Clust (strict)"("Visible"=w193) -> ()  [unwired: 2 in, 2 out]
            n113 = property on="On/Off" class="Bool (strict)"("Visible"=w193) -> ()  [unwired: 2 in, 2 out]
            n114 = property on="Test Slider" class="Slide (strict)"("Visible"=w193) -> ()  [unwired: 2 in, 2 out]
          }
          frame "Analog Out", "Motor", "PWM" {
            w199 = FALSE ("Visible")
            n115 = case shown="\"Analog Out\"" w198 {
              tunnel: [1.0 ("Value") -1.0 ("Value") 0.0 ("Value")] -> w197
              tunnel: [255.0 ("Value") 1.0 ("Value") 5.0 ("Value")] -> w196
              tunnel: [128.0 ("Value") 0.0 ("Value") 0.0 ("Value")] -> w195
              tunnel: [64.0 ("Value") 0.5 ("Value") 1.0 ("Value")] -> w194
              frame "PWM" {
              }
              frame "Motor", Default {
              }
              frame "Analog Out" {
              }
            }
            n116 = property on="Motor" class="Clust (strict)"("Visible"=TRUE) -> ()  [unwired: 2 in, 2 out]
            n117 = property on="Value" class="Slide (strict)"("Value"=w195, "Scale.Minimum"=w197, "Scale.Maximum"=w196, "Scale.Increment"=w194) -> ()  [unwired: 2 in, 2 out]
            n118 = property on="On/Off" class="Bool (strict)"("Visible"=w199) -> ()  [unwired: 2 in, 2 out]
            n119 = property on="Test Slider" class="Slide (strict)"("Visible"=w199) -> ()  [unwired: 2 in, 2 out]
            n120 = property on="Test Ring" class="Ring (strict)"("Visible"=w199) -> ()  [unwired: 2 in, 2 out]
            n121 = property on="Rev/Fwd" class="Clust (strict)"("Visible"=w199) -> ()  [unwired: 2 in, 2 out]
          }
          frame "Servo" {
            w215 = FALSE ("Visible")
            n122 = call <vilib>:"NT Read Number.vi"("name"=w217) -> ("value"=w216:dbl)  [unwired: 8 in, 2 out]
            n123 = property on="Test Slider" class="Slide (strict)"("Visible"=TRUE, "Scale.Maximum"=170.0 ("Scale.Range:Maximum")) -> ()  [unwired: 2 in, 2 out]
            n124 = local write "Test Slider"(w216) -> ()
            n125 = property on="Motor" class="Clust (strict)"("Visible"=w215) -> ()  [unwired: 2 in, 2 out]
            n126 = property on="Rev/Fwd" class="Clust (strict)"("Visible"=w215) -> ()  [unwired: 2 in, 2 out]
            n127 = property on="On/Off" class="Bool (strict)"("Visible"=w215) -> ()  [unwired: 2 in, 2 out]
            n128 = property on="Test Ring" class="Ring (strict)"("Visible"=w215) -> ()  [unwired: 2 in, 2 out]
          }
          frame "Relay", "Solenoid" {
            w218 = FALSE ("Visible")
            n129 = property on="Motor" class="Clust (strict)"("Visible"=w218) -> ()  [unwired: 2 in, 2 out]
            n130 = property on="Test Slider" class="Slide (strict)"("Visible"=w218) -> ()  [unwired: 2 in, 2 out]
            n131 = Search and Replace String(input string=w219, search string="/Value  **", replace string="/Direction") -> (result string=w225:string)  [unwired: 5 in, 3 out]
            n132 = property on="Test Ring" class="Ring (strict)"("Visible"=w218) -> ()  [unwired: 2 in, 2 out]
            n133 = call <vilib>:"NT Read String.vi"("name"=w225) -> ("value"=w223:string)  [unwired: 8 in, 2 out]
            n134 = Equal?(x="Both directions", y=w223) -> (x = y?=w221:bool)
            n135 = Not(x=w221) -> (.not. x?=w222:bool)
            n136 = property on="Rev/Fwd" class="Clust (strict)"("Visible"=w221) -> ()  [unwired: 2 in, 2 out]
            n137 = property on="On/Off" class="Bool (strict)"("Visible"=w222, "Caption.Text"=w220) -> ()  [unwired: 2 in, 2 out]
          }
          frame "Compressor", "Digital Out" {
            w228 = FALSE ("Visible")
            # "Get direction and finish"
            n138 = property on="Motor" class="Clust (strict)"("Visible"=w228) -> ()  [unwired: 2 in, 2 out]
            n139 = property on="Test Slider" class="Slide (strict)"("Visible"=w228) -> ()  [unwired: 2 in, 2 out]
            n140 = property on="Test Ring" class="Ring (strict)"("Visible"=w228) -> ()  [unwired: 2 in, 2 out]
            n141 = property on="On/Off" class="Bool (strict)"("Visible"=TRUE, "Caption.Text"=w229) -> ()  [unwired: 2 in, 2 out]
            n142 = property on="Rev/Fwd" class="Clust (strict)"("Visible"=FALSE) -> ()  [unwired: 2 in, 2 out]
          }
          frame "Camera" {
            n143 = call <vilib>:"NT_Get Last Path Segment.vi"("String in"=w236) -> ("String out"=w237:string)  [unwired: 10 in]
            n144 = property on="On/Off" class="Bool (strict)"("Visible"=FALSE) -> ()  [unwired: 2 in, 2 out]
            n145 = property on="Motor" class="Clust (strict)"("Visible"=FALSE) -> ()  [unwired: 2 in, 2 out]
            n146 = property on="Rev/Fwd" class="Clust (strict)"("Visible"=FALSE) -> ()  [unwired: 2 in, 2 out]
            n147 = case shown="\"White Balance  **\"" w237 {
              tunnel: w236 -> [w243 w252 w261 w270 w279 _ w285]
              tunnel: w235 -> [w241 w249 w258 w267 w276 _ _]
              frame "Size  **" {
                n148 = Index Array(array=w241) -> (element=w240:cluster{string[]})  [unwired: 1 in]
                n149 = call <vilib>:"NT Read String.vi"("name"=w243) -> ("value"=w242:string)  [unwired: 8 in, 2 out]
                n150 = Unbundle(w240) -> (w238:string[])
                n151 = Match First String(2:w238, 3:w242) -> (0:w239:i32)  [unwired: 1 out]
                n152 = property on="Test Ring" class="Ring (strict)"("Value"=w239, "Strings []"=w238) -> ()  [unwired: 2 in, 2 out]
                n153 = property on="Test Ring" class="Ring (strict)"("Visible"=TRUE) -> ()  [unwired: 2 in, 2 out]
                n154 = property on="Test Slider" class="Slide (strict)"("Visible"=FALSE) -> ()  [unwired: 2 in, 2 out]
              }
              frame "White Balance  **" {
                n155 = Index Array(array=w249, index=1) -> (element=w250:cluster{string[]})
                n156 = call <vilib>:"NT Read String.vi"("name"=w252) -> ("value"=w251:string)  [unwired: 8 in, 2 out]
                n157 = Unbundle(w250) -> (w247:string[])
                n158 = Match First String(2:w247, 3:w251) -> (0:w246:i32)  [unwired: 1 out]
                n159 = property on="Test Ring" class="Ring (strict)"("Value"=w246, "Strings []"=w247) -> ()  [unwired: 2 in, 2 out]
                n160 = property on="Test Ring" class="Ring (strict)"("Visible"=TRUE) -> ()  [unwired: 2 in, 2 out]
                n161 = property on="Test Slider" class="Slide (strict)"("Visible"=FALSE) -> ()  [unwired: 2 in, 2 out]
              }
              frame "Exposure  **" {
                n162 = Index Array(array=w258, index=2) -> (element=w259:cluster{string[]})
                n163 = call <vilib>:"NT Read String.vi"("name"=w261) -> ("value"=w260:string)  [unwired: 8 in, 2 out]
                n164 = Unbundle(w259) -> (w255:string[])
                n165 = Match First String(2:w255, 3:w260) -> (0:w256:i32)  [unwired: 1 out]
                n166 = property on="Test Ring" class="Ring (strict)"("Value"=w256, "Strings []"=w255) -> ()  [unwired: 2 in, 2 out]
                n167 = property on="Test Ring" class="Ring (strict)"("Visible"=TRUE) -> ()  [unwired: 2 in, 2 out]
                n168 = property on="Test Slider" class="Slide (strict)"("Visible"=FALSE) -> ()  [unwired: 2 in, 2 out]
              }
              frame "Exposure Priority  **" {
                n169 = Index Array(array=w267, index=3) -> (element=w268:cluster{string[]})
                n170 = call <vilib>:"NT Read String.vi"("name"=w270) -> ("value"=w269:string)  [unwired: 8 in, 2 out]
                n171 = Unbundle(w268) -> (w264:string[])
                n172 = Match First String(2:w264, 3:w269) -> (0:w265:i32)  [unwired: 1 out]
                n173 = property on="Test Ring" class="Ring (strict)"("Value"=w265, "Strings []"=w264) -> ()  [unwired: 2 in, 2 out]
                n174 = property on="Test Ring" class="Ring (strict)"("Visible"=TRUE) -> ()  [unwired: 2 in, 2 out]
                n175 = property on="Test Slider" class="Slide (strict)"("Visible"=FALSE) -> ()  [unwired: 2 in, 2 out]
              }
              frame "Color Enable  **" {
                n176 = Index Array(array=w276, index=4) -> (element=w277:cluster{string[]})
                n177 = call <vilib>:"NT Read String.vi"("name"=w279) -> ("value"=w278:string)  [unwired: 8 in, 2 out]
                n178 = Unbundle(w277) -> (w273:string[])
                n179 = Match First String(2:w273, 3:w278) -> (0:w274:i32)  [unwired: 1 out]
                n180 = property on="Test Ring" class="Ring (strict)"("Value"=w274, "Strings []"=w273) -> ()  [unwired: 2 in, 2 out]
                n181 = property on="Test Ring" class="Ring (strict)"("Visible"=TRUE) -> ()  [unwired: 2 in, 2 out]
                n182 = property on="Test Slider" class="Slide (strict)"("Visible"=FALSE) -> ()  [unwired: 2 in, 2 out]
              }
              frame Default {
                n183 = property on="Test Ring" class="Ring (strict)"("Visible"=FALSE) -> ()  [unwired: 2 in, 2 out]
                n184 = property on="Test Slider" class="Slide (strict)"("Visible"=FALSE) -> ()  [unwired: 2 in, 2 out]
              }
              frame "Brightness  **", "Color Level  **", "Compression  **", "FPS  **", "Sharpness  **" {
                n185 = call <vilib>:"NT Read Number.vi"("name"=w285) -> ("value"=w284:dbl)  [unwired: 8 in, 2 out]
                n186 = local write "Test Slider"(w284) -> ()
                n187 = property on="Test Slider" class="Slide (strict)"("Visible"=TRUE, "Scale.Maximum"=100.0 ("Scale.Range:Maximum")) -> ()  [unwired: 2 in, 2 out]
                n188 = property on="Test Ring" class="Ring (strict)"("Visible"=FALSE) -> ()  [unwired: 2 in, 2 out]
              }
            }
          }
        }
        n189 = property on="Progress" class="Clust (strict)"("Visible"=FALSE) -> ()  [unwired: 2 in, 2 out]
      }
      event "Test Name": Mouse Enter {
        # "Populate the ring with the list of tests"
        n190 = event-data() -> ()  [unwired: 1 in, 1 out]
        n191 = call <vilib>:"NT Read String Array.vi"("name"="TestMode/TestList" ("Name")) -> ("value"=w292:string[])  [unwired: 8 in, 2 out]
        n192 = Build Array (concatenate)("Select the test to run...", w292) -> (w291:string[])
        n193 = property on="Test Name" class="Ring (strict)"("Strings []"=w291) -> ()  [unwired: 2 in, 2 out]
      }
      event "Test Name": Value Change {
        w293 = FALSE ("Visible")
        # "Tell the robot the test name to run"
        n194 = event-data() -> ("NewVal"=w297:u16)  [unwired: 1 in]
        n195 = property on="Test Name" class="Ring (strict)"() -> ("Strings []"=w298:string[])  [unwired: 2 in, 2 out]
        n196 = local write "Progress"(T6 {"Test Progress"=0, "Test Progress Text"=""} ("Progress")) -> ()
        n197 = Index Array(array=w298, index=w297) -> (element=w296:string)
        n198 = call <vilib>:"NT Write String.vi"("value"=w296, "name"="TestMode/TestName" ("Name")) -> ()  [unwired: 9 in, 1 out]
        n199 = property on="Progress" class="Clust (strict)"("Visible"=TRUE) -> ()  [unwired: 2 in, 2 out]
        n200 = property on="Motor" class="Clust (strict)"("Visible"=w293) -> ()  [unwired: 2 in, 2 out]
        n201 = property on="Test Slider" class="Slide (strict)"("Visible"=w293) -> ()  [unwired: 2 in, 2 out]
        n202 = property on="On/Off" class="Bool (strict)"("Visible"=w293) -> ()  [unwired: 2 in, 2 out]
        n203 = property on="Rev/Fwd" class="Clust (strict)"("Visible"=w293) -> ()  [unwired: 2 in, 2 out]
        n204 = property on="Test Ring" class="Ring (strict)"("Visible"=w293) -> ()  [unwired: 2 in, 2 out]
      }
      event "Select Auto": Mouse Enter {
        # "Populate the combo box with the list of autonomous options"
        n205 = event-data() -> ()  [unwired: 1 in, 1 out]
        n206 = call <vilib>:"NT Read String Array.vi"("name"="Auto List" ("Name")) -> ("value"=w300:string[])  [unwired: 8 in, 2 out]
        n207 = property on="Select Auto" class="CmbBox"("Strings[]"=w300) -> ()  [unwired: 2 in, 2 out]
      }
      event "Select Auto": Value Change {
        # "User modified the Auto Selection. Write to NT variable so robot knows."
        n208 = event-data() -> ("NewVal"=w302:string)  [unwired: 1 in]
        n209 = call <vilib>:"NT Write String.vi"("value"=w302, "name"="Auto Selector" ("Name")) -> ()  [unwired: 9 in, 1 out]
      }
      event "CheckList": Double Click {
        # "Shift clears all"
        # "Update symbols on the listbox"
        n210 = event-data() -> ("PlatMods.Shift"=w304:bool, "Row"=w306:i32)  [unwired: 1 in]
        n211 = case shown="True" w304 {
          tunnel: w306 -> [w310 _]
          tunnel: 1 -> [w309 _]
          frame False {
            n212 = property on="CheckList" class="LstBox (strict)"() -> ("Item Symbols"=w308:i32[])  [unwired: 2 in, 2 out]
            n213 = Replace Array Subset(array=w308, new element=w309, index=w310) -> (w307:i32[])
            n214 = property on="CheckList" class="LstBox (strict)"("Item Symbols"=w307) -> ()  [unwired: 2 in, 2 out]
          }
          frame True {
            w311 = 0 ("Top Row")
            n215 = property on="CheckList" class="LstBox (strict)"() -> ("Number of Rows"=w313:u32)  [unwired: 2 in, 2 out]
            n216 = Initialize Array(0, w313) -> (w312:i32[])
            n217 = property on="CheckList" class="LstBox (strict)"("Top Row"=w311, "Value"=w311, "Item Symbols"=w312) -> ()  [unwired: 2 in, 2 out]
          }
        }
      }
      event "CheckList": Key Down {
        # "Update symbols on the listbox\nLeft and right keys check and uncheck"
        n218 = event-data() -> ("VKey"=w316:T22)  [unwired: 1 in]
        n219 = case shown="\"Left\", \"Right\"" w316 {
          selector: w316 -> [w321 _]
          tunnel: eventvkey."Left" ("VKey") -> [w319 _]
          frame "Left", "Right" {
            n220 = Equal?(x=w319, y=w321) -> (x = y?=w320:bool)
            n221 = Select(t=0, s=w320, f=1) -> (s? t:f=w322:i32)
            n222 = property on="CheckList" class="LstBox (strict)"() -> ("Item Symbols"=w325:i32[])  [unwired: 2 in, 2 out]
            n223 = Replace Array Subset(array=w325, new element=w322, index="CheckList") -> (w324:i32[])
            n224 = property on="CheckList" class="LstBox (strict)"("Item Symbols"=w324) -> ()  [unwired: 2 in, 2 out]
          }
          frame Default {
          }
        }
      }
      event "Motor.Enable": Value Change {
        # "When the test mode otor enable helper is set, update that\ntree row item's value"
        n225 = event-data() -> ("NewVal"=w330:bool)  [unwired: 1 in]
        n226 = Unbundle("Motor") -> ("Value"=w329:dbl)  [unwired: 1 out]
        n227 = Select(t=w329, s=w330, f=0.0) -> (s? t:f=w327:dbl)
        n228 = call <vilib>:"NT Write Number.vi"("value"=w327, "name"=w326) -> ()  [unwired: 9 in, 1 out]
      }
      event "Test Slider": Value Change {
        # "When the test mode slider helper is set, update that\ntree row item's value"
        n229 = event-data() -> ("NewVal"=w332:dbl)  [unwired: 1 in]
        n230 = call <vilib>:"NT Write Number.vi"("value"=w332, "name"=w333) -> ()  [unwired: 9 in, 1 out]
      }
      event "On/Off": Value Change {
        # "When the test mode on/off helper value is set, update that\ntree row item's value"
        n231 = event-data() -> ("NewVal"=w336:bool)  [unwired: 1 in]
        n232 = Boolean To (0,1)(Boolean=w336) -> (0, 1=w335:i16)
        n233 = call <vilib>:"NT Write Number.vi"("value"=w335, "name"=w334) -> ()  [unwired: 9 in, 1 out]
      }
      event "Rev/Fwd": Value Change {
        # "When the test mode helper value for relays is set, update that\ntree row item's value"
        n234 = event-data() -> ("NewVal.Forward"=w343:bool, "NewVal.Reverse"=w342:bool)  [unwired: 1 in]
        n235 = Boolean To (0,1)(Boolean=w343) -> (0, 1=w339:i16)
        n236 = Boolean To (0,1)(Boolean=w342) -> (0, 1=w341:i16)
        n237 = Negate(x=w341) -> (-x=w340:i16)
        n238 = Add(x=w339, y=w340) -> (x+y=w338:i16)
        n239 = call <vilib>:"NT Write Number.vi"("value"=w338, "name"=w337) -> ()  [unwired: 9 in, 1 out]
      }
      event "Test Ring": Value Change {
        # "When a test mode helper value is selected from the ring,\nset the tree item's variable to the string value"
        n240 = event-data() -> ("NewVal"=w346:u16)  [unwired: 1 in]
        n241 = property on="Test Ring" class="Ring (strict)"() -> ("Strings []"=w347:string[])  [unwired: 2 in, 2 out]
        n242 = Index Array(array=w347, index=w346) -> (element=w345:string)
        n243 = call <vilib>:"NT Write String.vi"("value"=w345, "name"=w344) -> ()  [unwired: 9 in, 1 out]
      }
      event "Rec Mode": Value Change {
        # "Update globals for recording mode and path to read log from.\nClear when logging and let NetworkTables set path for vision to\nuse."
        n244 = event-data() -> ("NewVal"=w356:enum32{"Stop", "Record", "Playback"})  [unwired: 1 in]
        n245 = global write "WPI_DashboardLogging Global.vi" "Logging Filename"(path "") -> ()
        n246 = global write "WPI_DashboardLogging Global.vi" "Recording"(w356) -> ()
        n247 = case shown="\"Playback\"" w356 {
          tunnel: w355 -> [_ w358 w366]
          tunnel: [_ _ w365] -> w353
          tunnel: [_ _ w364] -> _
          tunnel: w351 -> [_ _ w362]
          tunnel: cluster{i32, i32} {-250, 170} -> [_ _ w361]
          tunnel: [_ _ T23 {"Image Size"=TRUE, "Image Type"=TRUE, "Pixel Value"=TRUE, "ROI Information"=TRUE, "Zoom Factor"=FALSE} ("Image Information Shown:All Elements")] -> w348
          tunnel: [_ _ TRUE ("Zoom Factor")] -> w349
          frame Default {
          }
          frame "Stop", "Record" {
            # "Place Window too"
            n248 = invoke class="VI" method="FP.Close"(reference=w358) -> (reference out=w357:refnum<vi>)  [unwired: 2 in, 2 out]
            n249 = invoke class="VI" method="Abort VI"(reference=w357) -> ()  [unwired: 2 in, 3 out]
          }
          frame "Playback" {
            n250 = call "Open Playback Panel.vi"("Offset"=w361, "DB VI Ref"=w362, "Playback in"=w366) -> ("Playback out"=w363:refnum<vi>)  [unwired: 8 in]
            n251 = register-events(w363) -> (reference out=w365:refnum<event-registration>, error out=w364:errorcluster)  [unwired: 2 in]
          }
        }
        n252 = property on="Camera Image Right" class="ImageControl"("Image Information Shown"=w348, "Image Information Visible"=w349) -> ()  [unwired: 2 in, 2 out]
        n253 = property on="Camera Image" class="ImageControl"("Image Information Shown"=w348, "Image Information Visible"=w349) -> ()  [unwired: 2 in, 2 out]
        n254 = call <vilib>:"WPI_DashboardNT Log FieldName Cache.vi"("Operation"=enum16{"Lookup/Add", "Index", "Clear"}."Clear") -> ()  [unwired: 8 in, 3 out]
      }
      event Panel Close {
        w367 = enum32{"Stop", "Record", "Playback"}."Stop" ("Rec Mode")
        # "Playback window has been closed, abort"
        n255 = event-data() -> ()  [unwired: 1 in, 4 out]
        n256 = local write "Rec Mode"(w367) -> ()
        n257 = global write "WPI_DashboardLogging Global.vi" "Recording"(w367) -> ()
      }
      event Panel Close {
        # "Abort playback window and ourself"
        n258 = event-data() -> ()  [unwired: 1 in, 4 out]
        n259 = invoke class="VI" method="FP.Close"(reference=w370) -> (reference out=w369:refnum<vi>)  [unwired: 2 in, 2 out]
        n260 = invoke class="VI" method="Abort VI"(reference=w369) -> (error out=w368:errorcluster)  [unwired: 2 in, 2 out]
        n261 = invoke class="VI" method="Abort VI"(error in=w368) -> ()  [unwired: 2 in, 3 out]
      }
      event "Tree": Double Click {
        n262 = event-data() -> ("PlatMods"=w376:T25, "Tag"=w373:string)  [unwired: 1 in]
        n263 = Unbundle(w376) -> ("Shift"=w375:bool)  [unwired: 4 out]
        n264 = String Subset(string=w373, length (rest)=1 ("length (rest)")) -> (substring=w372:string)  [unwired: 1 in]
        n265 = Not(x=w375) -> (.not. x?=w374:bool)
        n266 = case shown="\"/\"" w372 {
          tunnel: w373 -> [_ w378]
          tunnel: w374 -> [_ w377]
          frame Default {
          }
          frame "/" {
            n267 = call <vilib>:"NT Update Persistence.vi"("Persistence"=w377, "Name"=w378) -> ()  [unwired: 9 in, 1 out]
          }
        }
      }
    }
  }
  n268 = while {
    tunnel: w54 -> [w380]
    i -> [w383]
    stop <- FALSE stop-if-true
    n269 = Wait (ms)(milliseconds to wait=u32 100) -> ()  [unwired: 1 out]
    n270 = case shown="\"Playback\"" "Rec Mode" {
      tunnel: w383 -> [_ _ w398]
      tunnel: [u32 2829099 ("Base Color") u32 11141120 ("Target Color") w387] -> w379
      frame "Stop", Default {
        # "Reset the color, extra updates don't cost much"
      }
      frame "Record" {
      }
      frame "Playback" {
        # "Playback"
        n271 = Quotient & Remainder(x=w398, y=u32 50 ("milliseconds to wait")) -> (x-y*floor(x/y)=w394:u32)  [unwired: 1 out]
        n272 = Divide(x=w394, y=u32 50 ("milliseconds to wait")) -> (x/y=w391:dbl)
        n273 = Multiply(x=6.283185307179586, y=w391) -> (x*y=w396:dbl)
        n274 = Sine(x=w396) -> (sin(x)=w395:dbl)
        n275 = Absolute Value(x=w395) -> (abs(x)=w388:dbl)
        n276 = call "Interpolate RGB Color.vi"("Proportion"=w388, "Target Color"=u32 30976, "Base Color"=u32 2829099) -> ("Result Color"=w387:u32)  [unwired: 8 in]
      }
    }
    n277 = property class="Pane"(reference=w380, "PaneColor"=w379) -> ()  [unwired: 1 in, 2 out]
  }
  n278 = local write "Dashboard Tab"(T2."Drive" ("Dashboard Tab")) -> ()
  n279 = property on="On/Off" class="Bool (strict)"("Visible"=w26) -> ()  [unwired: 2 in, 2 out]
  n280 = property on="Motor" class="Clust (strict)"("Visible"=w26) -> ()  [unwired: 2 in, 2 out]
  n281 = property on="Progress" class="Clust (strict)"("Visible"=w26) -> ()  [unwired: 2 in, 2 out]
  n282 = property on="Test Ring" class="Ring (strict)"("Visible"=w26) -> ()  [unwired: 2 in, 2 out]
  n283 = property on="Rev/Fwd" class="Clust (strict)"("Visible"=w26) -> ()  [unwired: 2 in, 2 out]
  n284 = while {
    tunnel: u16 1741 ("timeout ms (25000)") -> [w400]
    stop <- FALSE stop-if-true
    n285 = TCP Create Listener(10:w400) -> (0:w399:errorcluster, 3:w401:refnum<k5>)  [unwired: 4 in, 1 out]
    n286 = case shown="No Error" w399 {
      selector: w399 -> [w403 _]
      tunnel: w401 -> [w404 _]
      frame No Error {
        n287 = while {
          tunnel: w404 -> [w407]
          tunnel: w403 -> [w406]
          stop <- FALSE stop-if-true
          n288 = TCP Wait On Listener(8:w406, 11:w407) -> (0:w408:errorcluster, 4:w409:refnum<k5>)  [unwired: 2 in, 3 out]
          n289 = local write "TCP"(w409) -> ()
          n290 = case shown="Error" w408 {
            frame No Error {
            }
            frame Error {
              n291 = Wait (ms)(milliseconds to wait=u32 1000) -> ()  [unwired: 1 out]
            }
          }
        }
      }
      frame Error {
        n292 = Wait (ms)(milliseconds to wait=u32 1000) -> ()  [unwired: 1 out]
      }
    }
  }
  n293 = global write "WPI_DashboardLogging Global.vi" "Recording"(w49) -> ()
  n294 = local write "Rec Mode"(w49) -> ()
  n295 = call <vilib>:"NT Write String.vi"("value"="Select Auto", "name"="Auto Selector" ("Name")) -> ()  [unwired: 9 in, 1 out]
